vi "Network-Order Bytes To Words U8.vi"(1 "bytes in":u8[](array[numeric]) format="%02x") -> (0 "words out":u8[](array[numeric]) format="%x")   [LabVIEW 2020, in "NI_Bit Manipulation.lvlib"]
uses:
  <vilib>/Bit Manipulation/NI_Bit Manipulation.lvlib
  445b2e95-4c26-4098-854f-89dad29dbcf2.vi
  445b2e95-4c26-4098-854f-89dad29dbcf2.vi/19a10621-53ed-4da6-9507-4c1e7673ea65.vi
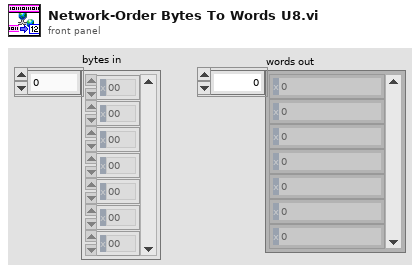
[diagram p1: front panel]
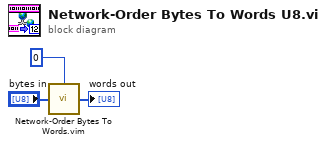
[diagram p0: block diagram]
diagram:
  n1 = call "Network-Order Bytes To Words.vim"("bytes in"="bytes in", "word type"=u8 0) -> ("words out"=→"words out":u8[])
